vi "ISM-Relay Toggle.vi"() -> ()   [LabVIEW 2011]
uses:
  <vilib>/LabVIEW Interface for Arduino/Type Defs/Pin Mode.ctl
  <vilib>/LabVIEW Interface for Arduino/LabVIEW Interface for Arduino.lvlib
panel:
  in  "Boolean":bool
  in  "Digital I/O Pin":u8=10
  in  "Relay Bit Pattern":u8=1 format="%x"
  in  "Stop":bool
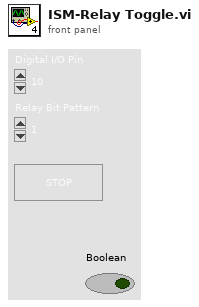
[diagram p1: front panel]
types:
  T1 = typedef "LabVIEW Interface for Arduino.lvlib/Pin Mode.ctl" = enum8{"Input", "Output"}
  T2 = typedef "LabVIEW Interface for Arduino.lvlib/Arduino Resource.ctl" = cluster{"VISA resource":refnum<visa-resource-name>, "Board Type":T3, "Connection Type":enum8{"USB / Serial"}, "Bytes Per Packet (15)":u8}
  T3 = typedef "LabVIEW Interface for Arduino.lvlib/Board Type.ctl" = enum16{"Uno", "Dimuelanove w/Atmega 328", "Mega 2560"}
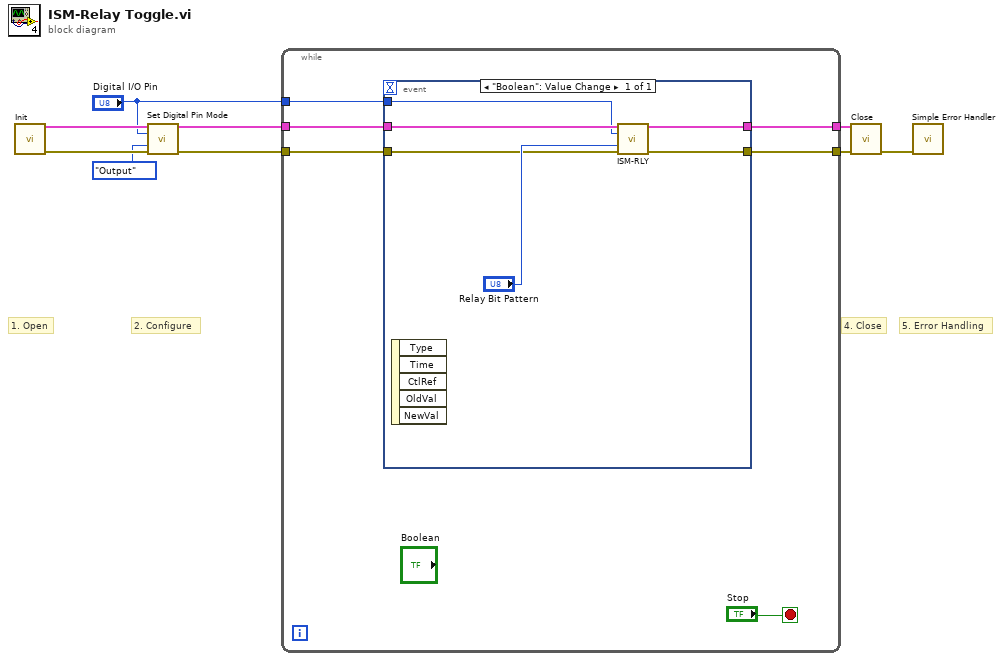
[diagram p0: block diagram]
diagram:
  # "5. Error Handling"
  # "4. Close"
  # "2. Configure"
  # "1. Open"
  n1 = call <vilib>:"Init.vi"() -> ("Arduino Resource"=w6:T2, "error out"=w5:errorcluster)  [unwired: 18 in]
  n2 = call <vilib>:"Set Digital Pin Mode.vi"("Arduino Resource"=w6, "Digital I/O Pin"="Digital I/O Pin", "Pin Mode (Input)"=Pin_Mode."Output", "error in"=w5) -> ("Arduino Resource"=w4:T2, "error out"=w3:errorcluster)  [unwired: 10 in]
  n3 = while {
    tunnel: [w13] -> w8
    tunnel: w4 -> [w14]
    tunnel: w3 -> [w12]
    tunnel: [w10] -> w7
    tunnel: "Digital I/O Pin" -> [w11]
    stop <- "Stop" stop-if-true
    n4 = event shown="[0] \"Boolean\": Value Change" {
      selector: _ -> [_]
      dyn-events: _ -> [_]
      timeout: _ -> [_]
      tunnel: w14 -> [w21]
      tunnel: [w20] -> w13
      tunnel: w12 -> [w18]
      tunnel: w11 -> [w17]
      tunnel: [w16] -> w10
      event "Boolean": Value Change {
        n5 = event-data() -> ()  [unwired: 1 in, 5 out]
        n6 = call "ISM-RLY.vi"("Arduino Resource"=w21, "ISM Relay Card (CS)"=w17, "Value (0)"="Relay Bit Pattern", "error in"=w18) -> ("Arduino Resource"=w20:T2, "error out"=w16:errorcluster)  [unwired: 10 in]
      }
    }
  }
  n7 = call <vilib>:"Close.vi"("Arduino Resource"=w8, "error in"=w7) -> ("error out"=w9:errorcluster)  [unwired: 13 in]
  n8 = call <vilib>:"Simple Error Handler.vi"("error in (no error)"=w9) -> ()  [unwired: 4 in, 5 out]
